vi "niP2P Library Name.vi"() -> (0 "nip2p libname":path=path "nip2p.*")   [LabVIEW 2010]
doc: "Retrieve the correct name of the NI-P2P library based on the operating system."
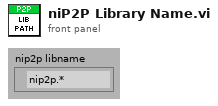
[diagram p1: front panel]
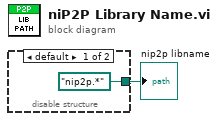
[diagram p0: block diagram]
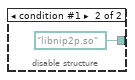
[diagram p2: hidden frame]
diagram:
  n1 = disable-structure shown="default" {
    disable-tunnel: [path "nip2p.*" ("path in") path "libnip2p.so" ("path in")] -> w1
    frame condition #0 (active) {
    }
    frame condition #1 {
    }
  }
  "nip2p libname" <- w1
